vi "Read Binary Config.vi"(4 "Class Name is Included":bool, 6 "byte order (0:big-endian, network order)":T1(ring), 8 "error in (no error)":errorcluster, 10 "Binary":string, 11 "abs_SharedVar_Bool in":refnum<class "conc_SharedVar_I16.lvclass">) -> (0 "error out":errorcluster, 2 "Remaining":string, 3 "abs_SharedVar_Bool out":refnum<class "conc_SharedVar_I16.lvclass">)   [LabVIEW 2021, in "conc_SharedVar_I16.lvclass"]
doc: "LVabs_Shared Variable 1.0.0.2\nTim - TSA\nCopyright (c) 2024, TSA"
uses:
  conc_SharedVar_I16.lvclass
  conc_SharedVar_I16.lvclass/conc_SharedVar_I16.ctl
  <vilib>/TSA/Abstract Data Classes/Abs_Types/I16 Integer/Abs_I16 Integer.lvclass
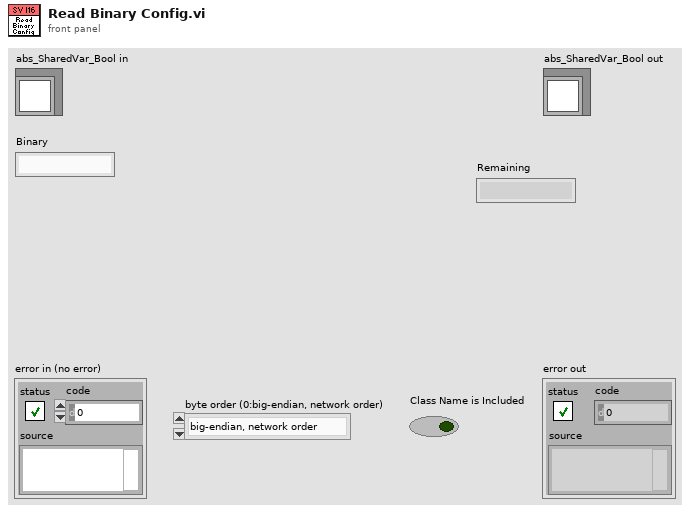
[diagram p1: front panel]
types:
  T1 = enum16{"big-endian, network order", "native, host order", "little-endian"}
  T2 = cluster{"Shared Variable Refnum":refnum<k21>, "Write Access":enum8{"Allowed", "Required", "None"}, "Read Access":enum8{"Allowed", "Required", "None"}}
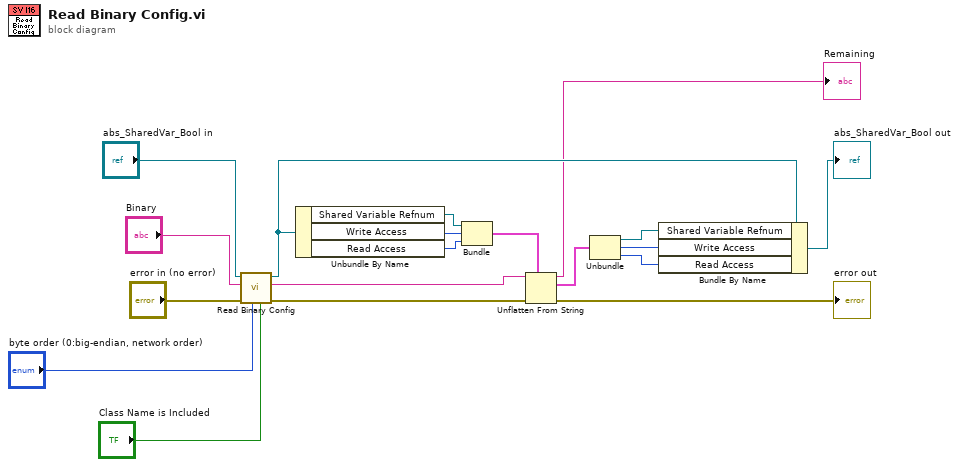
[diagram p0: block diagram]
diagram:
  n1 = call-parent "Read Binary Config.vi"("Class Name is Included"="Class Name is Included", "byte order (0:big-endian, network order)"="byte order (0:big-endian, network order)", "error in (no error)"="error in (no error)", "Binary"="Binary", "Abs_Type in"="abs_SharedVar_Bool in") -> ("error out"=w11:errorcluster, "Remaining"=w10:string, "Abs_Type out"=w7:refnum<class "conc_SharedVar_I16.lvclass">)  [unwired: 4 in]
  n2 = Unbundle By Name(w7) -> ("Shared Variable Refnum"=w14:refnum<k21>, "Write Access"=w13:enum8{"Allowed", "Required", "None"}, "Read Access"=w12:enum8{"Allowed", "Required", "None"})
  n3 = Bundle("Shared Variable Refnum"=w14, "Write Access"=w13, "Read Access"=w12) -> (w9:T2)  [unwired: 1 in]
  n4 = Unflatten From String(type=w9, binary string=w10, error in (no error)=w11) -> (rest of the binary string=→"Remaining":string, value=w5:T2, error out=→"error out":errorcluster)  [unwired: 2 in]
  n5 = Unbundle(w5) -> ("Shared Variable Refnum"=w4:refnum<k21>, "Write Access"=w3:enum8{"Allowed", "Required", "None"}, "Read Access"=w2:enum8{"Allowed", "Required", "None"})
  n6 = Bundle By Name(cluster=w7, "Shared Variable Refnum"=w4, "Write Access"=w3, "Read Access"=w2) -> (→"abs_SharedVar_Bool out":refnum<class "conc_SharedVar_I16.lvclass">)
